vi "atcs_getEvent_RejectedCommand.vi"(8 "error in (no error)":errorcluster, 11 "logevent_RejectedCommand_Ctl":T1) -> (0 "error out":errorcluster, 2 "function return":i32, 3 "logevent_RejectedCommand_Ctl out":T1)   [LabVIEW 2016, in "SALLV_atcs.lvlib"]
doc: "int atcs_shm_getEvent_RejectedCommandLV(atcs_logevent_RejectedCommandLV *logevent_RejectedCommand_Ctl );"
uses:
  SALLV_atcs.lvlib
  DataTypes/logevent_RejectedCommand.ctl
  SALLV_atcs.so
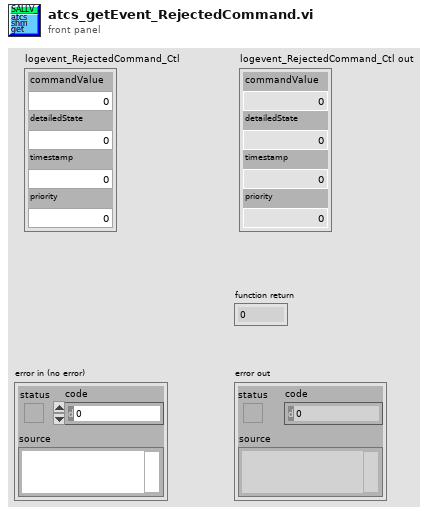
[diagram p1: front panel]
types:
  T1 = typedef "SALLV_atcs.lvlib/logevent_RejectedCommand.ctl" = cluster{"commandValue":i16, "detailedState":i32, "timestamp":dbl, "priority":i32}
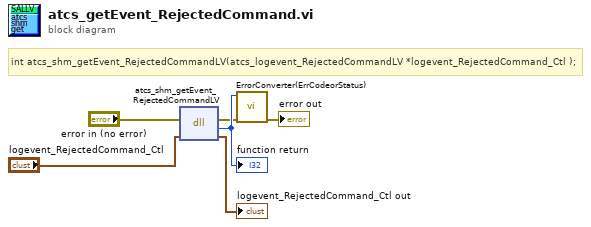
[diagram p0: block diagram]
diagram:
  # "int atcs_shm_getEvent_RejectedCommandLV(atcs_logevent_RejectedCommandLV *logevent_RejectedCommand_Ctl );"
  n1 = dll-call lib="home/andres/Desktop/SALLV_atcs/SALLV_atcs.*" fn="atcs_shm_getEvent_RejectedCommandLV"(error in="error in (no error)", "logevent_RejectedCommand_Ctl"="logevent_RejectedCommand_Ctl") -> (error out=w2:errorcluster, w6:i32, "logevent_RejectedCommand_Ctl"=→"logevent_RejectedCommand_Ctl out":T1)  [unwired: 2 in, 1 out]
  "function return" <- w6
  n2 = call "ErrorConverter(ErrCodeorStatus).vi"("error in (no error)"=w2, "error code"=w6) -> ("error out"=→"error out":errorcluster)  [unwired: 9 in]
